vi "MSEncoder Case-2-Stop.vi"(8 "error in (no error)":errorcluster, 11 "MSEncoder in":refnum<class "MSEncoder.lvclass">) -> (0 "error out":errorcluster, 3 "MSEncoder out":refnum<class "MSEncoder.lvclass">)   [LabVIEW 2018, in "MSEncoder.lvclass"]
uses:
  MSEncoder.lvclass
  MSEncoder.lvclass/MSEncoder.ctl
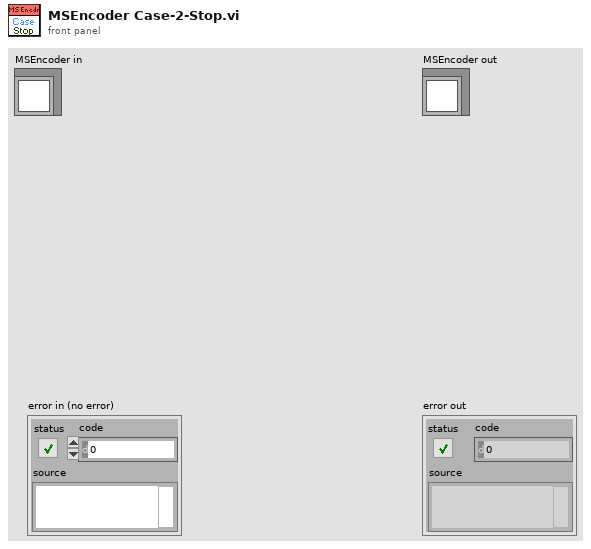
[diagram p1: front panel]
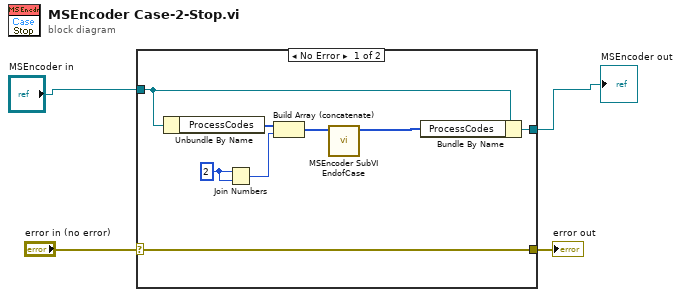
[diagram p0: block diagram]
diagram:
  n1 = case shown="No Error" "error in (no error)" {
    selector: "error in (no error)" -> [w11 w14]
    tunnel: "MSEncoder in" -> [w10 w13]
    tunnel: [w11 w14] -> w3
    tunnel: [w9 w13] -> w2
    frame No Error {
      w8 = u32 2
      n2 = Unbundle By Name(w10) -> ("ProcessCodes"=w12:u64[])
      n3 = Join Numbers(hi=w8, lo=w8) -> ((hi.lo)=w7:u64)
      n4 = Build Array (concatenate)(w12, w7) -> (w6:u64[])
      n5 = call "MSEncoder SubVI EndofCase.vi"("Case codes"=w6) -> ("Case codes with end"=w5:u64[])  [unwired: 9 in, 1 out]
      n6 = Bundle By Name(cluster=w10, "ProcessCodes"=w5) -> (w9:refnum<class "MSEncoder.lvclass">)
    }
    frame Error {
    }
  }
  "error out" <- w3
  "MSEncoder out" <- w2
